vi "binding_path.vi"() -> (0 "appended path":path)   [LabVIEW 2022 SP3]
panel:
  in  "name or relative path":path=path "labview_splitted.py"
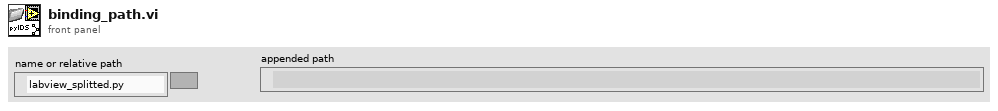
[diagram p1: front panel]
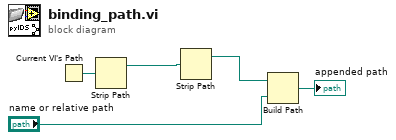
[diagram p0: block diagram]
diagram:
  n1 = Current VI's Path() -> (path=w3:path)
  n2 = Strip Path(path=w3) -> (stripped path=w2:path)  [unwired: 1 out]
  n3 = Strip Path(path=w2) -> (stripped path=w1:path)  [unwired: 1 out]
  n4 = Build Path(base path=w1, name or relative path="name or relative path") -> (appended path=→"appended path":path)
